vi "2 Compares.vi"(0 "InA I32":i32, 5 "InA DBL":dbl, 7 "Select A/B":bool, 9 "InB I32":i32, 11 "InB DBL":dbl) -> (6 "Out I32":i32, 10 "Out DBL":dbl)   [LabVIEW 2010]
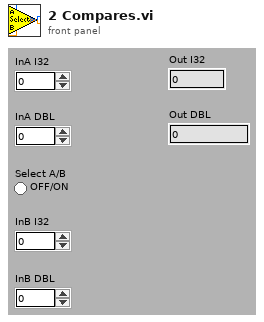
[diagram p1: front panel]
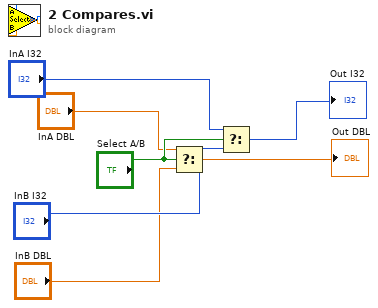
[diagram p0: block diagram]
diagram:
  n1 = Select(t="InA DBL", s="Select A/B", f="InB DBL") -> (s? t:f=→"Out DBL":dbl)
  n2 = Select(t="InA I32", s="Select A/B", f="InB I32") -> (s? t:f=→"Out I32":i32)
